vi "Untitl 1.vi"() -> ()   [LabVIEW 2020]
panel:
  in  "?":bool
  out "Signal":dynamicdata(graph)
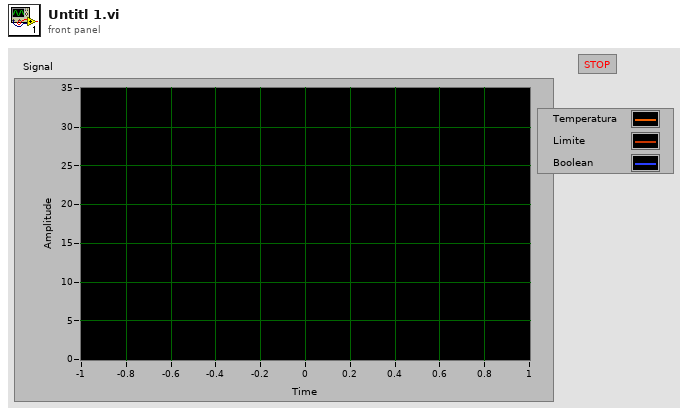
[diagram p1: front panel]
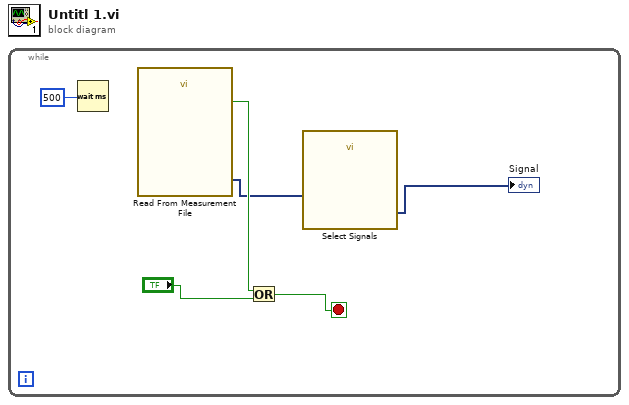
[diagram p0: block diagram]
diagram:
  n1 = while {
    stop <- w5 stop-if-true
    n2 = Wait (ms)(milliseconds to wait=500) -> ()  [unwired: 1 out]
    n3 = call "Read From Measurement File"() -> ("Signals"=w2:dynamicdata, "EOF?"=w3:bool)  [unwired: 6 in, 4 out]
    n4 = Or(x=w3, y="?") -> (x .or. y?=w5:bool)
    n5 = call "Select Signals"("Signals"=w2) -> ("Signal Out"=→"Signal":dynamicdata)  [unwired: 9 in, 1 out]
  }
